vi "Diagnostics Substate Complete_UI.vi"(8 "error in (no error)":errorcluster, 10 "Diagnostics Completion\nSubstate cluster in":T1={"Diagnostics Successful?"=TRUE, "Popup/Status String"=""}, 11 "ZenGage v3.0 UI in":refnum<class "ZenGage v3.0 UI.lvclass">) -> (0 "error out":errorcluster, 3 "ZenGage v3.0 UI out":refnum<class "ZenGage v3.0 UI.lvclass">)   [LabVIEW 2015, in "ZenGage v3.0 UI.lvclass"]
uses:
  ZenGage v3.0 UI.lvclass
  Type Definitions/Diagnostics/Diagnostics Done_Diagnostics_UI.ctl
  ZenGage v3.0 UI.lvclass/ZenGage v3.0 UI.ctl
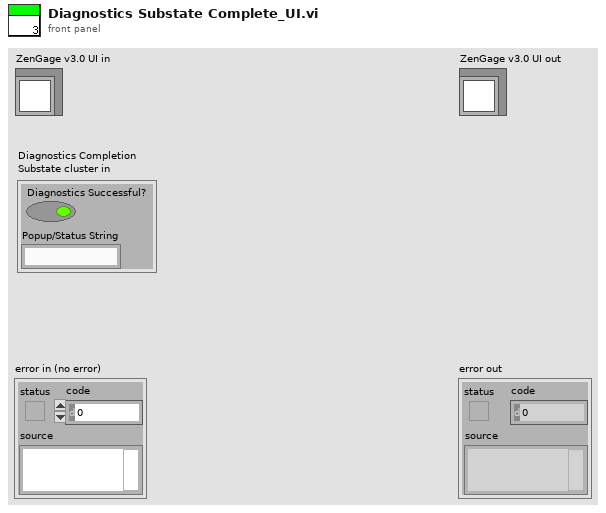
[diagram p1: front panel]
types:
  T1 = typedef "ZenGage v3.0 UI.lvclass/Diagnostics Done_Diagnostics_UI.ctl" = cluster{"Diagnostics Successful?":bool, "Popup/Status String":string}
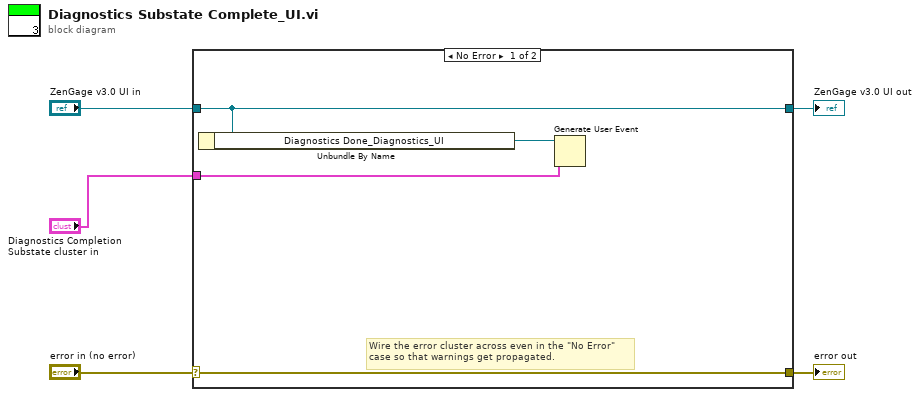
[diagram p0: block diagram]
diagram:
  n1 = case shown="No Error" "error in (no error)" {
    selector: "error in (no error)" -> [w9 w11]
    tunnel: [w9 w11] -> w4
    tunnel: [w8 w10] -> w2
    tunnel: "ZenGage v3.0 UI in" -> [w8 w10]
    tunnel: "Diagnostics Completion\nSubstate cluster in" -> [w6 _]
    frame No Error {
      # "Wire the error cluster across even in the \"No Error\"\ncase so that warnings get propagated."
      n2 = Unbundle By Name(w8) -> ("Diagnostics Done_Diagnostics_UI"=w7:refnum<user-event>)
      n3 = Generate User Event(user event=w7, event data cluster=w6) -> ()  [unwired: 2 in, 2 out]
    }
    frame Error {
    }
  }
  "error out" <- w4
  "ZenGage v3.0 UI out" <- w2
